vi "save.vi"(8 "error in (no error)":errorcluster, 11 "Notebook in":refnum<class "Notebook.lvclass">) -> (0 "error out":errorcluster, 3 "Notebook out":refnum<class "Notebook.lvclass">)   [LabVIEW 2010, in "Notebook.lvclass"]
uses:
  Notebook.lvclass
  Notebook.lvclass/Notebook.ctl
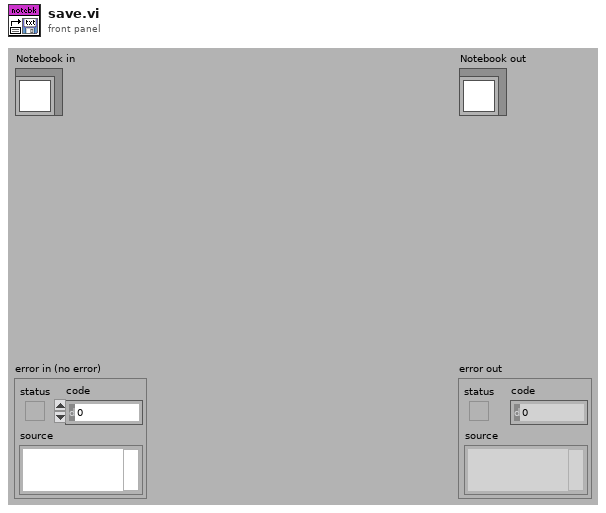
[diagram p1: front panel]
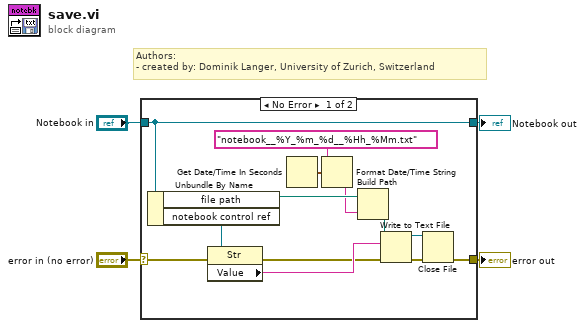
[diagram p0: block diagram]
diagram:
  # "Authors: \n- created by: Dominik Langer, University of Zurich, Switzerland"
  n1 = case shown="No Error" "error in (no error)" {
    selector: "error in (no error)" -> [w16 w19]
    tunnel: [w15 w19] -> w3
    tunnel: [w17 w18] -> w1
    tunnel: "Notebook in" -> [w17 w18]
    frame No Error {
      n2 = Unbundle By Name(w17) -> ("file path"=w7:path, "notebook control ref"=w14:refnum<vi>)
      n3 = property class="Str"(reference=w14, error in=w16) -> (error out=w12:errorcluster, "Value"=w13:string)  [unwired: 1 out]
      n4 = Get Date/Time In Seconds() -> (seconds since 1Jan1904=w9:timestamp)
      n5 = Format Date/Time String(time format string (%c)="notebook__%Y_%m_%d__%Hh_%Mm.txt", seconds (now)=w9) -> (date/time string=w6:string)  [unwired: 1 in]
      n6 = Build Path(base path=w7, name or relative path=w6) -> (appended path=w5:path)
      n7 = Write to Text File(file (use dialog)=w5, text=w13, error in=w12) -> (refnum out=w10:refnum<file>, error out=w11:errorcluster)  [unwired: 2 out]
      n8 = Close File(refnum=w10, error in=w11) -> (error out=w15:errorcluster)  [unwired: 1 out]
    }
    frame Error {
    }
  }
  "error out" <- w3
  "Notebook out" <- w1
